vi "Create LogFilepath.vi"(8 "error in (no error)":errorcluster, 10 "Log Directory":path, 11 "LogFile Type":T1) -> (0 "error out":errorcluster, 3 "Logfile Path":path)   [LabVIEW 2009]
uses:
  LogFileType.ctl
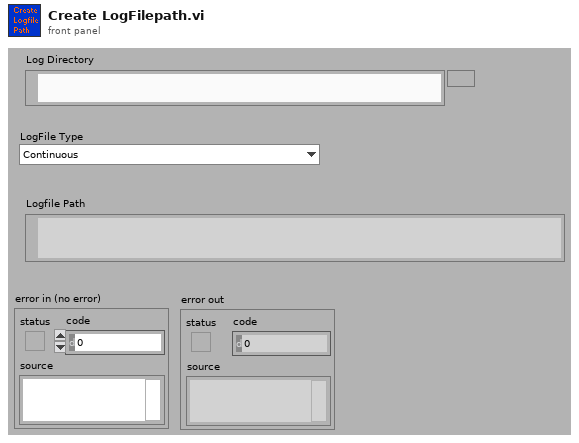
[diagram p1: front panel]
types:
  T1 = typedef "LogFileType.ctl" = enum16{"Continuous", "Step", "Volts", "Offsets", "Mixed Mode State", "DLL  Errors", "Snapshot", "End List"}
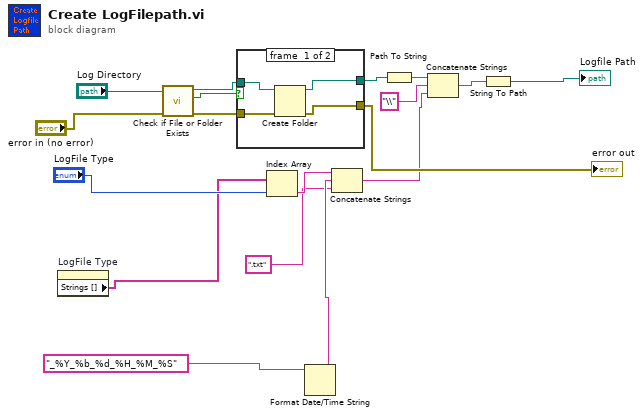
[diagram p0: block diagram]
diagram:
  n1 = property on="LogFile Type" class="Enum (strict)"() -> ("Strings []"=w1:string[])  [unwired: 2 in, 2 out]
  n2 = call <vilib>:"Check if File or Folder Exists.vi"("error in (no error)"="error in (no error)", "path"="Log Directory") -> ("error out"=w14:errorcluster, "file or folder exists?"=w15:bool, "dup path"=w16:path)  [unwired: 7 out]
  n3 = case shown="True" w15 {
    tunnel: w16 -> [w22 w24]
    tunnel: w14 -> [w21 w23]
    tunnel: [w20 w24] -> w12
    tunnel: [w19 w23] -> w6
    frame #0 {
      n4 = Create Folder(path (use dialog)=w22, error in=w21) -> (created path=w20:path, error out=w19:errorcluster)  [unwired: 2 out]
    }
    frame #1 {
    }
  }
  "error out" <- w6
  n5 = Index Array(array=w1, index="LogFile Type") -> (element=w10:string)
  n6 = Format Date/Time String(time format string (%c)="_%Y_%b_%d_%H_%M_%S") -> (date/time string=w9:string)  [unwired: 2 out]
  n7 = Concatenate Strings(w10, w9, ".txt" ("string")) -> (w3:string)
  n8 = Path To String(path=w12) -> (string=w5:string)
  n9 = Concatenate Strings(w5, "\\", w3) -> (w7:string)
  n10 = String To Path(string=w7) -> (path=→"Logfile Path":path)
